vi "Warp Affine (Greyscale).vi"(4 "Border Colour (Default: 0)":u8, 5 "Boarder Type (Default: DEFAULT)":T2=enum."DEFAULT", 6 "Required Destination Size":T5, 7 "Interpolation Mode (Default: CUBIC)":T4=enum."CUBIC", 8 "error in (no error)":errorcluster, 9 "2x3 Affine Matrix":T1, 10 "Greyscale Destination Image":T3, 11 "Greyscale Source Image":T3) -> (0 "error out":errorcluster, 3 "Greyscale Destination Image (duplicate)":T3)   [LabVIEW 2020, in "image.lvlib"]
uses:
  image.lvlib
  Greyscale Image.ctl
  common/Image Size (Integer).ctl
  Interpolation Mode.ctl
  Border Type.ctl
  <vilib>/Analysis/Matrix/Datatypes/RealMatrix.ctl
  b7e6b07f-7daf-4958-9fc0-179f1836a141.vi
  b7e6b07f-7daf-4958-9fc0-179f1836a141.vi/0c263cf4-9042-4d44-b92e-dafa676e1650.vi
  common/Module Path.vi
  <vilib>/Utility/error.llb/Error Cluster From Error Code.vi
  common/common.lvlib
  <vilib>/Analysis/Matrix/NI_Matrix.lvlib
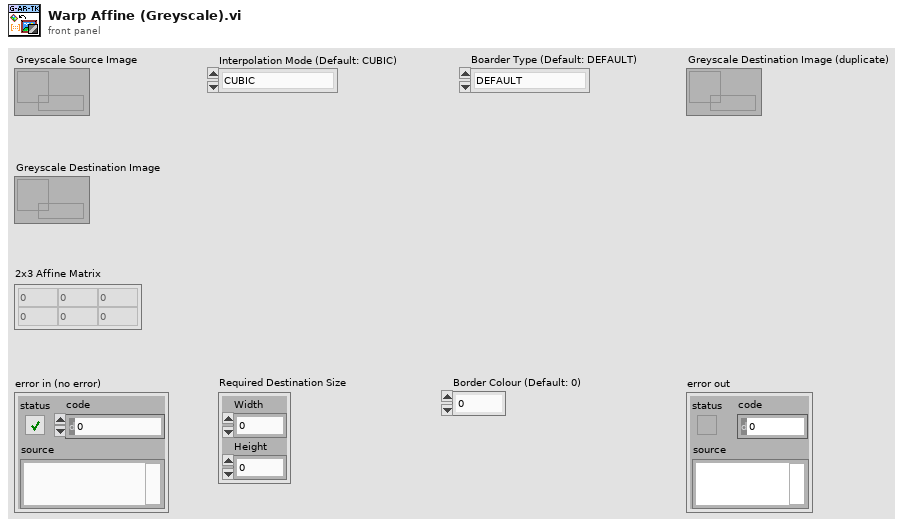
[diagram p1: front panel]
types:
  T1 = typedef "NI_Matrix.lvlib/RealMatrix.ctl" = dbl[][]
  T2 = typedef "image.lvlib/Border Type.ctl" = enum8{"CONSTANT", "REPLICATE", "REFLECT", "WRAP", "TRANSPARENT", "DEFAULT", "ISOLATED"}
  T3 = typedef "image.lvlib/Greyscale Image.ctl" = refnum<data-value>
  T4 = typedef "image.lvlib/Interpolation Mode.ctl" = enum8{"NEAREST", "LINEAR", "CUBIC", "AREA", "LANCZOS", "LINEAR_EXACT", "NEAREST_EXACT", "MAX"}
  T5 = typedef "common.lvlib/Image Size (Integer).ctl" = cluster{"Width":u16, "Height":u16}
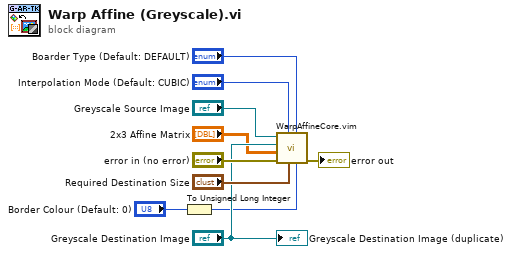
[diagram p0: block diagram]
diagram:
  n1 = To Unsigned Long Integer(number="Border Colour (Default: 0)") -> (unsigned 32bit integer=w1:u32)
  n2 = call "WarpAffineCore.vim"("Border Colour"=w1, "Boarder Type"="Boarder Type (Default: DEFAULT)", "Destination Size"="Required Destination Size", "Interpolation Mode"="Interpolation Mode (Default: CUBIC)", "error in (no error)"="error in (no error)", "Affine"="2x3 Affine Matrix", "Dst"="Greyscale Destination Image", "Src"="Greyscale Source Image") -> ("error out"=→"error out":errorcluster)  [unwired: 3 in]
  "Greyscale Destination Image (duplicate)" <- "Greyscale Destination Image"
